vi "Info.vi"(11 "Config Lookup in":refnum<class "Config Lookup.lvclass">) -> (1 "Meta":T1[](array[typedef]), 2 "Name":string)   [LabVIEW 2020, in "CDM-Config.lvlib" / "Config Lookup.lvclass"]
uses:
  Config Filter/Config Lookup.lvclass
  Meta Data.ctl
  Config Filter/Config Lookup.lvclass/Config Lookup.ctl
  CDM-Config.lvlib
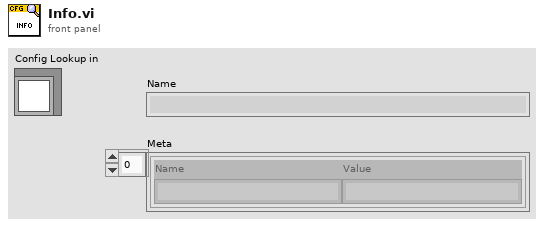
[diagram p1: front panel]
types:
  T1 = typedef "CDM-Config.lvlib/Meta Data.ctl" = cluster{"Name":string, "Value":string}
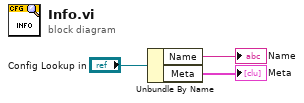
[diagram p0: block diagram]
diagram:
  n1 = Unbundle By Name("Config Lookup in") -> ("Name"=→"Name":string, "Meta"=→"Meta":T1[])
